vi "WriteTree.vi"(8 "error in":errorcluster, 11 "SystemConfigRepo in":refnum<class "SystemConfigRepo.lvclass">) -> (0 "error out":errorcluster, 2 "root":T1, 3 "repository out":refnum<class "NISE_CEF_Repository.lvclass">)   [LabVIEW 2013, in "PL Framework Configuration Tool.lvlib" / "SystemConfigRepo.lvclass"]
uses:
  SystemConfigRepo.lvclass
  <vilib>/NI/CEF/CEF_TreeControl/Repository/NISE_CEF_Repository.lvclass
  <vilib>/NI/CEF/CEF_TreeControl/Node/NodeRef.ctl
  <vilib>/NI/CEF/CEF_TreeControl/Node/NISE_CEF_Node.lvclass
  Systems/Systems.lvclass
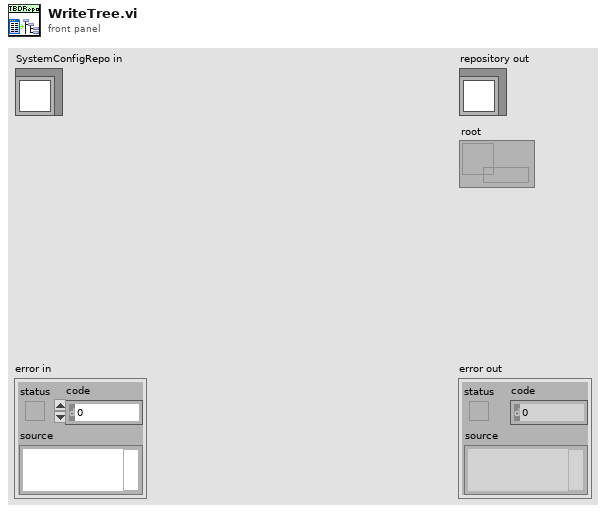
[diagram p1: front panel]
types:
  T1 = typedef "NISE_CEF_Node.lvclass/NodeRef.ctl" = refnum<data-value>
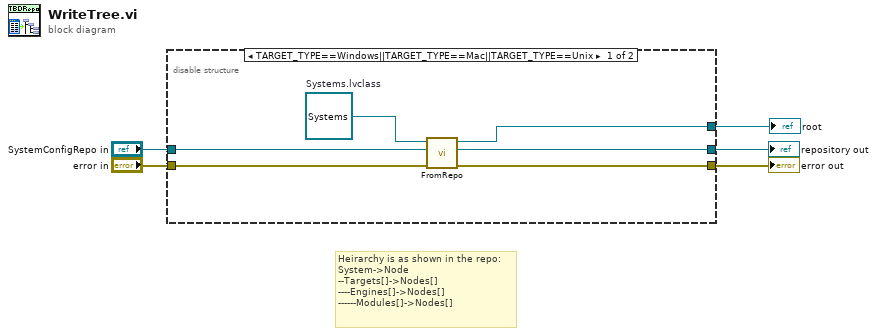
[diagram p0: block diagram]
diagram:
  # "Heirarchy is as shown in the repo:\nSystem->Node\n--Targets[]->Nodes[]\n----Engines[]->Nodes[]\n------Modules[]->Nodes[]"
  n1 = disable-structure shown="TARGET_TYPE==Windows||TARGET_TYPE==Mac||TARGET_TYPE==Unix" {
    disable-tunnel: "SystemConfigRepo in" -> [w10 w13]
    disable-tunnel: "error in" -> [w9 w12]
    disable-tunnel: [w8 w12] -> w3
    disable-tunnel: [w7 w13] -> w2
    disable-tunnel: [w6 _] -> w1
    frame condition #0 (active) {
      w11 = refnum<class "Systems.lvclass"> refnum  # Systems.lvclass
      n2 = call-dynamic "FromRepo.vi"("error in"=w9, "repository in"=w10, "Systems in"=w11) -> ("error out"=w8:errorcluster, "repository out"=w7:refnum<class "NISE_CEF_Repository.lvclass">, "node"=w6:T1)  [unwired: 6 in]
    }
    frame condition #1 {
    }
  }
  "error out" <- w3
  "repository out" <- w2
  "root" <- w1
